vi "Zach n' Zac Box.vi"(10 "JoystickDevRef":T1) -> (0 "Intake Deploy State":bool, 1 "Intake Motor Speed":dbl, 2 "Percent of Maximum Shooter RPM":dbl, 3 "Loader Motor Speed":dbl, 4 "Short Range?":bool, 6 "Long Range?":bool)   [LabVIEW 2011]
uses:
  <vilib>/Rock Robotics/WPI/Joystick/WPI_JoystickDevRef.ctl
  <vilib>/Rock Robotics/WPI/Joystick/WPI_JoystickDeviceEnum.ctl
panel:
  in  "ENABLE EMULATOR":bool
  in  "percent motor output":dbl(knob) scale=0.2..0.8
  in  "BUTTON 7":bool
  in  "BUTTON 5":bool
  in  "BUTTON 2":bool
  in  "Intake":bool
  out "Ball Loader State":bool
  # "This only overrides the % motor"
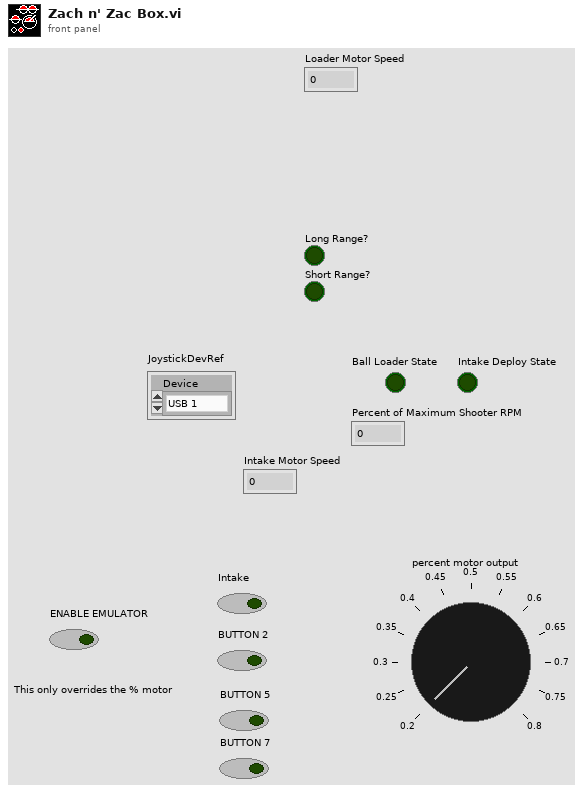
[diagram p1: front panel]
types:
  T1 = typedef "WPI_JoystickDevRef.ctl" = cluster{"Device":T2}
  T2 = typedef "WPI_JoystickDeviceEnum.ctl" = enum16{"USB 1", "USB 2", "USB 3", "USB 4", "Kinect 1", "Kinect 2"}
  T3 = typedef "WPI_JoystickButtonState.ctl" = cluster{"Button 1":bool, "Button 2":bool, "Button 3":bool, "Button 4":bool, "Button 5":bool, "Button 6":bool, "Button 7":bool, "Button 8":bool, "Button 9":bool, "Button 10":bool, "Button 11":bool, "Button 12":bool}
  T4 = cluster{"axis 1 (x)":dbl, "axis 2 (y)":dbl, "axis 3 (throttle)":dbl, "axis 4":dbl, "axis 5":dbl, "axis 6":dbl}
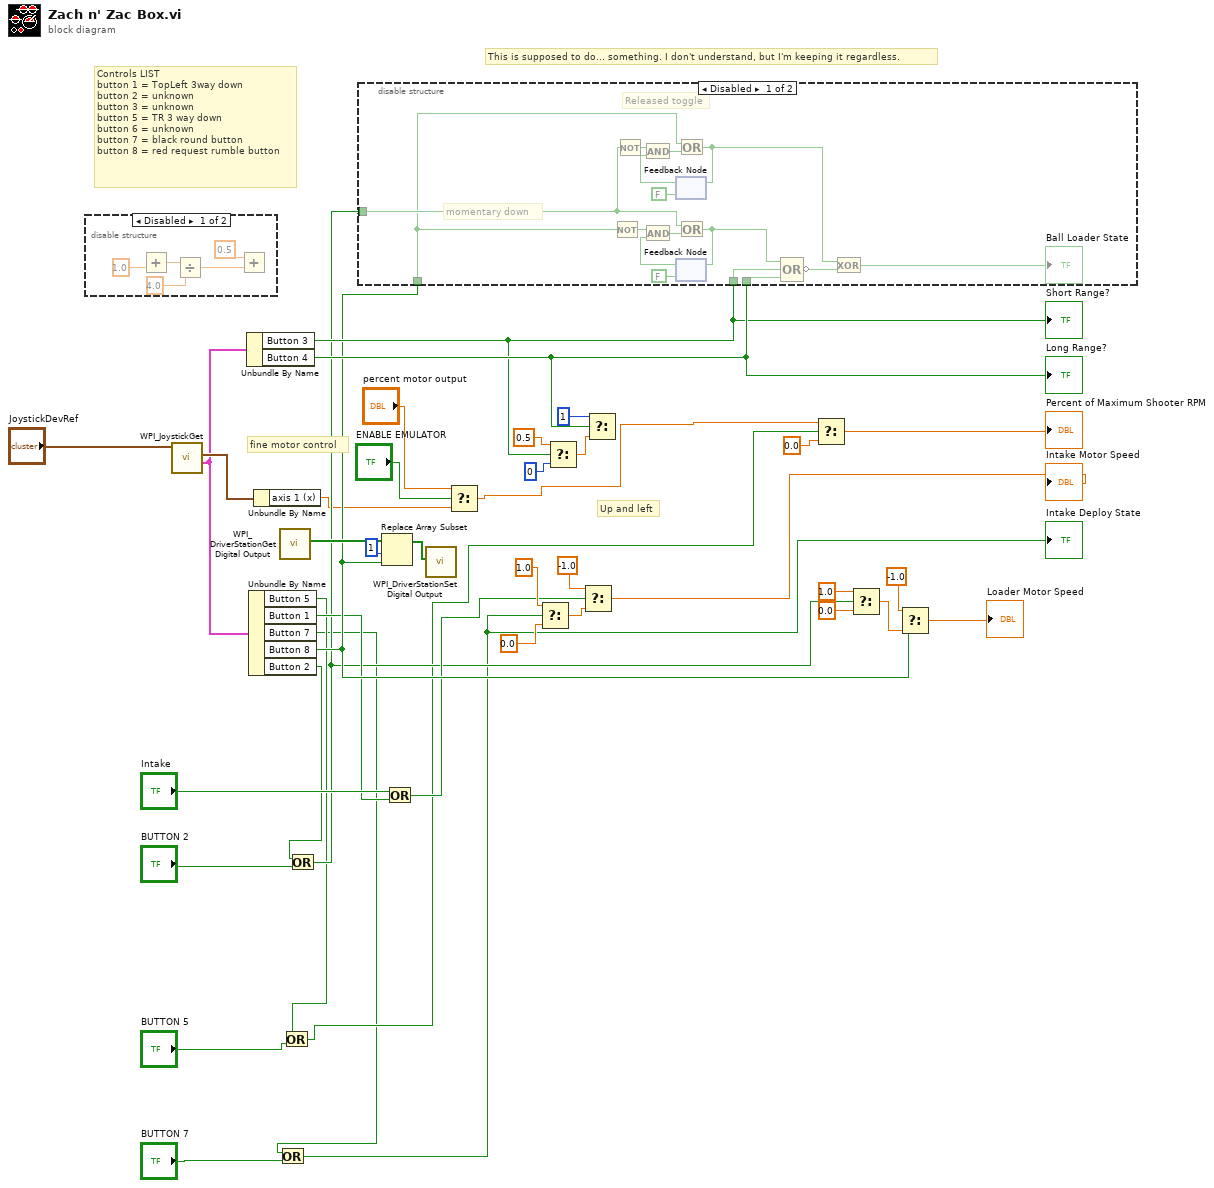
[diagram p0: block diagram]
diagram:
  # "Up and left"
  # "This is supposed to do... something. I don't understand, but I'm keeping it regardless."
  # "Controls LIST\nbutton 1 = TopLeft 3way down\nbutton 2 = unknown\nbutton 3 = unknown\nbutton 5 = TR 3 way down\nbutton 6 = unknown\nbutton 7 = black round button\nbutton 8 = red request rumble button"
  # "fine motor control"
  n1 = disable-structure shown="Disabled" {
    frame Disabled {
      n2 = Add(y=1.0) -> (x+y=w45:dbl)  [unwired: 1 in]
      n3 = Divide(x=w45, y=4.0) -> (x/y=w43:dbl)
      n4 = Add(x=0.5, y=w43) -> ()  [unwired: 1 out]
    }
    frame Enabled {
    }
  }
  n5 = call <vilib>:"WPI_JoystickGet.vi"("JoystickDevRef"="JoystickDevRef") -> ("Buttons"=w40:T3, "Axes"=w41:T4)  [unwired: 4 in, 1 out]
  n6 = Unbundle By Name(w40) -> ("Button 3"=w37:bool, "Button 4"=w38:bool)
  "Long Range?" <- w38
  "Short Range?" <- w37
  n7 = Unbundle By Name(w40) -> ("Button 5"=w7:bool, "Button 1"=w12:bool, "Button 7"=w6:bool, "Button 8"=w17:bool, "Button 2"=w9:bool)
  n8 = Unbundle By Name(w41) -> ("axis 1 (x)"=w3:dbl)
  n9 = Or(x=w6, y="BUTTON 7") -> (x .or. y?=w5:bool)
  "Intake Deploy State" <- w5
  n10 = call <vilib>:"WPI_DriverStationGet Digital Output.vi"() -> ("Driver Station Digital Output (1-8)"=w32:bool[])  [unwired: 10 in, 1 out]
  n11 = Or(x=w7, y="BUTTON 5") -> (x .or. y?=w8:bool)
  n12 = Or(x=w9, y="BUTTON 2") -> (x .or. y?=w10:bool)
  n13 = disable-structure shown="Disabled" {
    disable-tunnel: w38 -> [w51 _]
    disable-tunnel: w37 -> [w50 _]
    disable-tunnel: w10 -> [w48 _]
    disable-tunnel: w17 -> [w47 _]
    frame Disabled {
      # "momentary down"
      # "Released toggle"
      n14 = Not(x=w47) -> (.not. x?=w56:bool)
      n15 = Not(x=w48) -> (.not. x?=w55:bool)
      n16 = feedback #1(FALSE) -> (w57:bool)
      n17 = And(x=w55, y=w57) -> (x .and. y?=w58:bool)
      n18 = feedback #2(FALSE) -> (w60:bool)
      n19 = And(x=w56, y=w60) -> (x .and. y?=w61:bool)
      n20 = Or(x=w47, y=w58) -> (x .or. y?=w53:bool)
      n21 = feedback-in #1(w53) -> ()
      n22 = Or(x=w48, y=w61) -> (x .or. y?=w54:bool)
      n23 = feedback-in #2(w54) -> ()
      n24 = Compound Arithmetic op=OR(w54, w50, w51) -> (invert w52:bool)
      n25 = Exclusive Or(1:w52, 2:w53) -> (0:→"Ball Loader State":bool)
    }
    frame Enabled {
    }
  }
  n26 = Replace Array Subset(array=w32, new element=w17, index=1) -> (w30:bool[])
  n27 = Or(x="Intake", y=w12) -> (x .or. y?=w11:bool)
  n28 = call <vilib>:"WPI_DriverStationSet Digital Output.vi"("Driver Station Digital Output (1-8)"=w30) -> ()  [unwired: 10 in, 1 out]
  n29 = Select(t="percent motor output", s="ENABLE EMULATOR", f=w3) -> (s? t:f=w1:dbl)
  n30 = Select(t=1.0 ("y"), s=w5, f=0.0 ("y")) -> (s? t:f=w33:dbl)
  n31 = Select(t=0.5, s=w37, f=0) -> (s? t:f=w39:dbl)
  n32 = Select(t=-1.0 ("y"), s=w11, f=w33) -> (s? t:f=→"Intake Motor Speed":dbl)
  n33 = Select(t=1, s=w38, f=w39) -> ()  [unwired: 1 out]
  n34 = Select(t=w1, s=w8, f=0.0) -> (s? t:f=→"Percent of Maximum Shooter RPM":dbl)
  n35 = Select(t=1.0, s=w10, f=0.0) -> (s? t:f=w24:dbl)
  n36 = Select(t=-1.0, s=w17, f=w24) -> (s? t:f=→"Loader Motor Speed":dbl)
